vi "Set Log File Reference.vi"(8 "Error In":errorcluster, 10 "Log File Reference":refnum<file>, 11 "Error Handling In":refnum<class "Error Handling.lvclass">) -> (0 "Error Out":errorcluster, 3 "Error Handling Out":refnum<class "Error Handling.lvclass">)   [LabVIEW 2021, in "Error Handling.lvclass"]
uses:
  Error Handling.lvclass
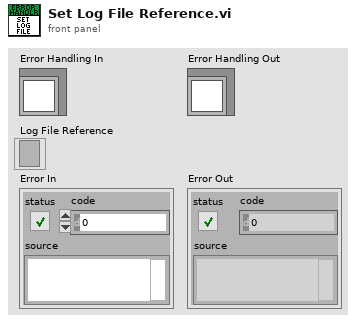
[diagram p1: front panel]
types:
  T1 = typedef "Error Handling.lvclass/Data.ctl" = cluster{"Log File Reference":refnum<file>}
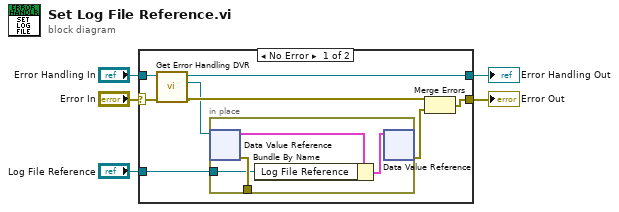
[diagram p0: block diagram]
diagram:
  n1 = case shown="No Error" "Error In" {
    selector: "Error In" -> [w9 w18]
    tunnel: [w12 w18] -> w2
    tunnel: [w8 w19] -> w5
    tunnel: "Error Handling In" -> [w10 w19]
    tunnel: "Log File Reference" -> [w11 _]
    frame No Error {
      n2 = call "Get Error Handling DVR.vi"("Error In"=w9, "Error Handling In"=w10) -> ("Error Out"=w7:errorcluster, "DVR"=w6:refnum<data-value>, "Error Handling Out"=w8:refnum<class "Error Handling.lvclass">)  [unwired: 7 in]
      n3 = in-place {
        in-place-border: [w17] -> _
        in-place-border: w11 -> [w14]
        n4 = in-place-dvr #1(w6) -> (w16:T1, w17:errorcluster)
        n5 = Bundle By Name(cluster=w16, "Log File Reference"=w14) -> (w15:T1)
        n6 = in-place-dvr #1(w15) -> (w13:errorcluster)  [unwired: 1 out]
      }
      n7 = Merge Errors(w7, w13) -> (w12:errorcluster)
    }
    frame Error {
    }
  }
  "Error Handling Out" <- w5
  "Error Out" <- w2
